vi "Send Manual Operation.vi"(0 "VISA resource name":refnum<visa-resource-name>, 5 "Channel (0001)":string="0001", 7 "Manual Operation Type (0 : Execute Alarm Acknowledge)":i32(ring) items=["Execute Alarm Acknowledge", "Execute Manual Sampling", "Activate Manual Trigger", "Take a Snapshot", "Forced Timeout of The Display Data", "Forced Timeout of The Event Data", "Execute Individual Alarm Acknowledge"], 9 "Alarm Number (1)":i32=1 min=1 max=4 step=1, 11 "error in (no error)":errorcluster) -> (4 "VISA resource name out":refnum<visa-resource-name>, 15 "error out":errorcluster)   [LabVIEW 2020, in "Yokogawa GX Series.lvlib"]
doc: "This VI runs manual operation that alarm acknowledge, manual sample, manual trigger, snapshot, forced timeout of the display data or forced timeout of the event data."
uses:
  <instrlib>/Yokogawa GX Series/Yokogawa GX Series.lvlib
panel:
  in  "Batch Group Number  (0: OFF)":i32(ring) items=["OFF", "1", "2", "3", "4", "5", "6", "7", "8", "9", "10", "11", "12", "ALL"]
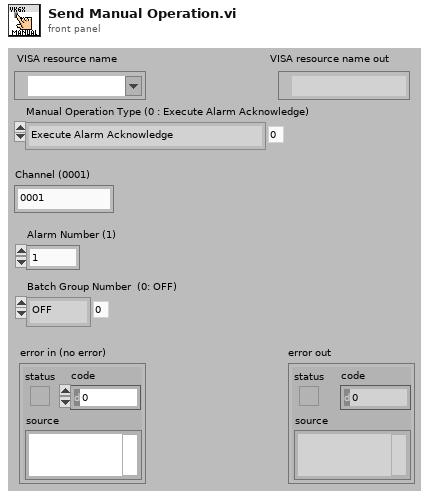
[diagram p1: front panel]
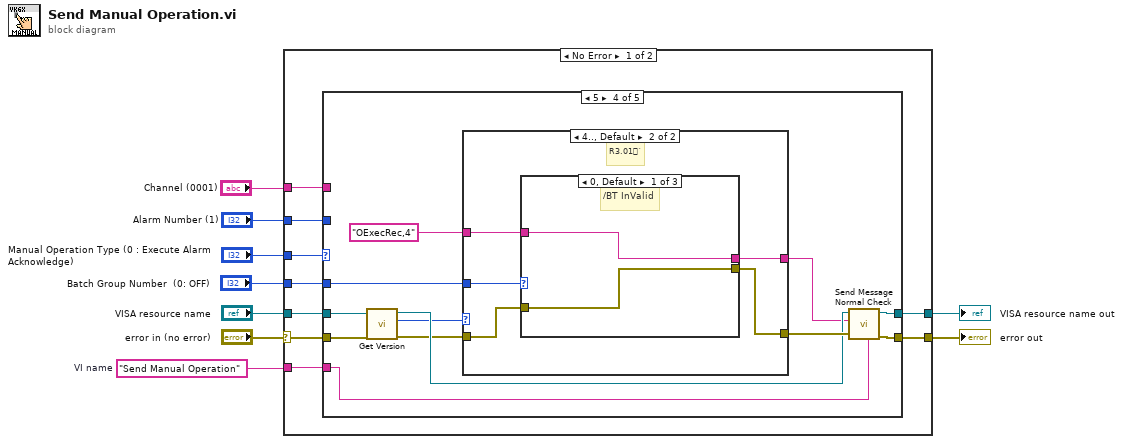
[diagram p0: block diagram]
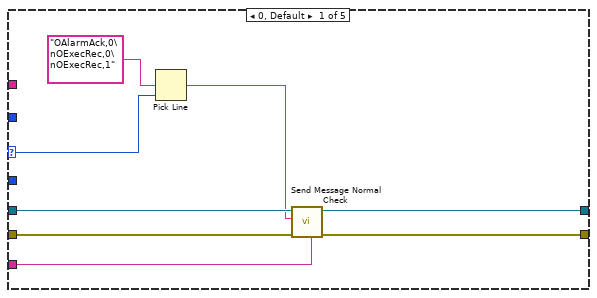
[diagram p2: hidden frame]
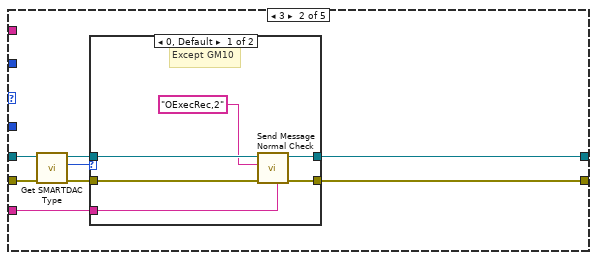
[diagram p3: hidden frame]
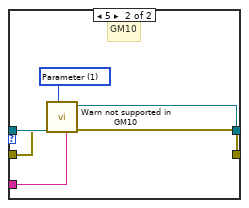
[diagram p4: hidden frame]
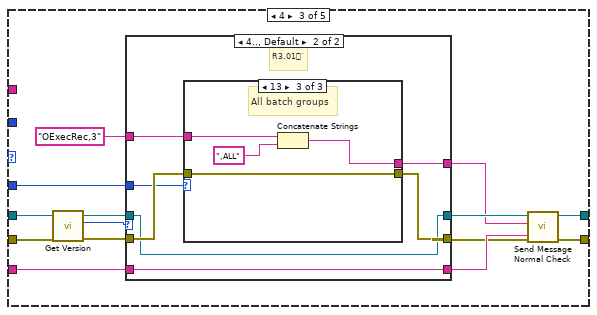
[diagram p5: hidden frame]
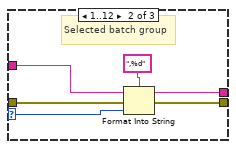
[diagram p8: hidden frame]
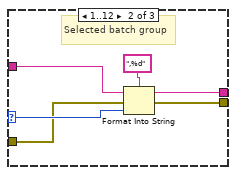
[diagram p10: hidden frame]
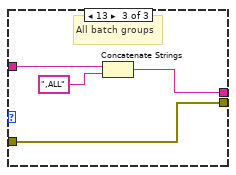
[diagram p11: hidden frame]
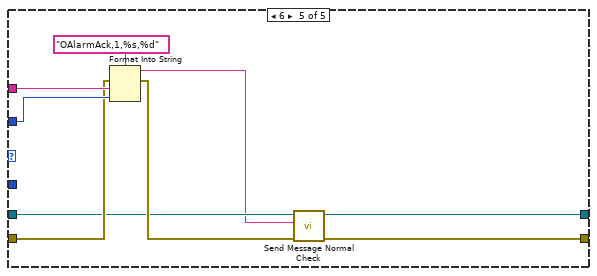
[diagram p12: hidden frame]
diagram:
  w7 = "Send Manual Operation"  # VI name
  n1 = case shown="No Error" "error in (no error)" {
    selector: "error in (no error)" -> [w15 w124]
    tunnel: "Manual Operation Type (0 : Execute Alarm Acknowledge)" -> [w18 _]
    tunnel: "VISA resource name" -> [w13 w125]
    tunnel: w7 -> [w14 _]
    tunnel: [w12 w125] -> w6
    tunnel: [w11 w124] -> w5
    tunnel: "Channel (0001)" -> [w17 _]
    tunnel: "Alarm Number (1)" -> [w16 _]
    tunnel: "Batch Group Number  (0: OFF)" -> [w10 _]
    frame No Error {
      n2 = case shown="5" w18 {
        selector: w18 -> [w25 _ _ _ _]
        tunnel: w17 -> [_ _ _ _ w122]
        tunnel: w16 -> [_ _ _ _ w121]
        tunnel: w15 -> [w23 w30 w55 w92 w120]
        tunnel: w14 -> [w19 w32 w60 w89 _]
        tunnel: w13 -> [w24 w31 w56 w93 w118]
        tunnel: [w21 w34 w59 w95 w116] -> w12
        tunnel: [w20 w33 w58 w94 w115] -> w11
        tunnel: w10 -> [_ _ w47 w86 _]
        frame 0, Default {
          n3 = Pick Line(multi-line string="OAlarmAck,0\nOExecRec,0\nOExecRec,1", line index=w25) -> (output string=w22:string)  [unwired: 1 out]
          n4 = call <instrlib>:"Send Message Normal Check.vi"("Source (\"\")"=w19, "error in (no error)"=w23, "Send Message (\"\")"=w22, "VISA resource name"=w24) -> ("error out"=w20:errorcluster, "VISA resource name out"=w21:refnum<visa-resource-name>)  [unwired: 2 in, 4 out]
        }
        frame 3 {
          n5 = call <instrlib>:"Get SMARTDAC Type.vi"("error in (no error)"=w30, "VISA resource name"=w31) -> ("error out"=w29:errorcluster, "SMARTDAC+ Type"=w28:u16, "VISA resource name out"=w27:refnum<visa-resource-name>)  [unwired: 7 in]
          n6 = case shown="0, Default" w28 {
            tunnel: [w40 w43] -> w34
            tunnel: [w39 w42] -> w33
            tunnel: w27 -> [w38 w45]
            tunnel: w29 -> [w37 w44]
            tunnel: w32 -> [w35 w41]
            frame 0, Default {
              # "Except GM10"
              n7 = call <instrlib>:"Send Message Normal Check.vi"("Source (\"\")"=w35, "error in (no error)"=w37, "Send Message (\"\")"="OExecRec,2", "VISA resource name"=w38) -> ("error out"=w39:errorcluster, "VISA resource name out"=w40:refnum<visa-resource-name>)  [unwired: 2 in, 4 out]
            }
            frame 5 {
              w46 = u16 1 items=["Command", "Parameter"] ("Kind (0: Command)")
              # "GM10"
              n8 = call <instrlib>:"Warn not supported in GM10.vi"("Source (\"\")"=w41, "Kind (0: Command)"=w46, "error in (no error)"=w44, "VISA resource name"=w45) -> ("error out"=w42:errorcluster, "VISA resource name out"=w43:refnum<visa-resource-name>)  [unwired: 6 in]
            }
          }
        }
        frame 4 {
          n9 = call <instrlib>:"Get Version.vi"("error in (no error)"=w55, "VISA resource name"=w56) -> ("error out"=w50:errorcluster, "Version"=w54:i32, "VISA resource name out"=w52:refnum<visa-resource-name>)  [unwired: 7 in]
          n10 = case shown="4.., Default" w54 {
            tunnel: w60 -> [w61 w71]
            tunnel: "OExecRec,3" -> [w64 w70]
            tunnel: [w63 w65] -> w53
            tunnel: w52 -> [w63 w65]
            tunnel: [w61 w71] -> w51
            tunnel: w50 -> [w62 w68]
            tunnel: [w62 w67] -> w49
            tunnel: [w64 w69] -> w48
            tunnel: w47 -> [_ w66]
            frame 0..3 {
              # "R1.03,R2.02,R2.03"
            }
            frame 4.., Default {
              # "R3.01`"
              n11 = case shown="13" w66 {
                selector: w66 -> [_ w74 _]
                tunnel: w70 -> [w73 w78 w83]
                tunnel: w68 -> [w72 w77 w80]
                tunnel: [w72 w76 w80] -> w67
                tunnel: [w73 w75 w82] -> w69
                frame 0, Default {
                  # "/BT InValid"
                }
                frame 1..12 {
                  # "Selected batch group"
                  n12 = Format Into String(format string=",%d", initial string=w78, error in=w77, w74) -> (resulting string=w75:string, error out=w76:errorcluster)
                }
                frame 13 {
                  # "All batch groups"
                  n13 = Concatenate Strings(w83, ",ALL") -> (w82:string)
                }
              }
            }
          }
          n14 = call <instrlib>:"Send Message Normal Check.vi"("Source (\"\")"=w51, "error in (no error)"=w49, "Send Message (\"\")"=w48, "VISA resource name"=w53) -> ("error out"=w58:errorcluster, "VISA resource name out"=w59:refnum<visa-resource-name>)  [unwired: 2 in, 4 out]
        }
        frame 5 {
          n15 = call <instrlib>:"Get Version.vi"("error in (no error)"=w92, "VISA resource name"=w93) -> ("error out"=w87:errorcluster, "Version"=w88:i32, "VISA resource name out"=w90:refnum<visa-resource-name>)  [unwired: 7 in]
          n16 = case shown="4.., Default" w88 {
            tunnel: [w96 w101] -> w91
            tunnel: [w97 w102] -> w84
            tunnel: w87 -> [w96 w100]
            tunnel: w86 -> [_ w99]
            tunnel: "OExecRec,4" -> [w97 w98]
            frame 0..3 {
              # "R1.03,R2.02,R2.03"
            }
            frame 4.., Default {
              # "R3.01`"
              n17 = case shown="0, Default" w99 {
                selector: w99 -> [_ w107 _]
                tunnel: [w103 w109 w112] -> w101
                tunnel: [w104 w108 w114] -> w102
                tunnel: w100 -> [w103 w105 w112]
                tunnel: w98 -> [w104 w106 w111]
                frame 0, Default {
                  # "/BT InValid"
                }
                frame 1..12 {
                  # "Selected batch group"
                  n18 = Format Into String(format string=",%d", initial string=w106, error in=w105, w107) -> (resulting string=w108:string, error out=w109:errorcluster)
                }
                frame 13 {
                  # "All batch groups"
                  n19 = Concatenate Strings(w111, ",ALL") -> (w114:string)
                }
              }
            }
          }
          n20 = call <instrlib>:"Send Message Normal Check.vi"("Source (\"\")"=w89, "error in (no error)"=w91, "Send Message (\"\")"=w84, "VISA resource name"=w90) -> ("error out"=w94:errorcluster, "VISA resource name out"=w95:refnum<visa-resource-name>)  [unwired: 2 in, 4 out]
        }
        frame 6 {
          n21 = Format Into String(format string="OAlarmAck,1,%s,%d", error in=w120, w122, w121) -> (resulting string=w117:string, error out=w119:errorcluster)  [unwired: 1 in]
          n22 = call <instrlib>:"Send Message Normal Check.vi"("error in (no error)"=w119, "Send Message (\"\")"=w117, "VISA resource name"=w118) -> ("error out"=w115:errorcluster, "VISA resource name out"=w116:refnum<visa-resource-name>)  [unwired: 3 in, 4 out]
        }
      }
    }
    frame Error {
    }
  }
  "error out" <- w5
  "VISA resource name out" <- w6
